vi "Write 7z config.vi"(8 "error in (no error)":errorcluster, 11 "PostBuildSupport in":refnum<class "PostBuildSupport.lvclass">) -> (0 "error out":errorcluster, 3 "PostBuildSupport out":refnum<class "PostBuildSupport.lvclass">)   [LabVIEW 2019, in "PostBuildSupport.lvclass"]
uses:
  PostBuildSupport.lvclass
  PostBuildSupport.lvclass/PostBuildSupport.ctl
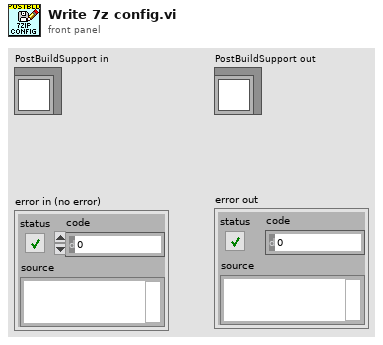
[diagram p1: front panel]
types:
  T1 = enum16{"open", "replace", "create", "open or create", "replace or create", "replace or create with confirmation"}
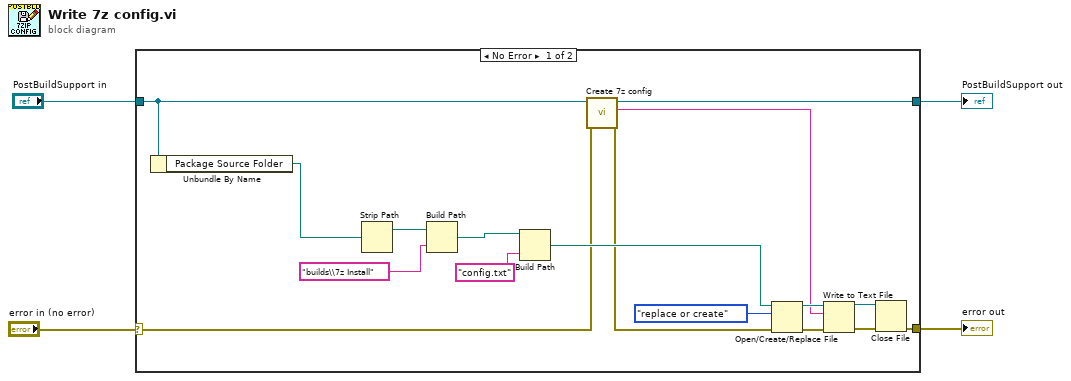
[diagram p0: block diagram]
diagram:
  n1 = case shown="No Error" "error in (no error)" {
    selector: "error in (no error)" -> [w9 w22]
    tunnel: [w13 w22] -> w4
    tunnel: "PostBuildSupport in" -> [w5 w23]
    tunnel: [w6 w23] -> w2
    frame No Error {
      n2 = Unbundle By Name(w5) -> ("Package Source Folder"=w10:path)
      n3 = Strip Path(path=w10) -> (stripped path=w20:path)  [unwired: 1 out]
      n4 = Build Path(base path=w20, name or relative path="builds\\7z Install") -> (appended path=w12:path)
      n5 = Build Path(base path=w12, name or relative path="config.txt") -> (appended path=w17:path)
      n6 = call "Create 7z config.vi"("error in (no error)"=w9, "PostBuildSupport in"=w5) -> ("error out"=w8:errorcluster, "resulting string"=w7:string, "PostBuildSupport out"=w6:refnum<class "PostBuildSupport.lvclass">)  [unwired: 7 in]
      n7 = Open/Create/Replace File(file path (use dialog)=w17, error in=w8, operation (0:open)=T1."replace or create") -> (refnum out=w19:refnum<file>, error out=w18:errorcluster)  [unwired: 3 in, 1 out]
      n8 = Write to Text File(file (use dialog)=w19, text=w7, error in=w18) -> (refnum out=w14:refnum<file>, error out=w15:errorcluster)  [unwired: 1 in, 1 out]
      n9 = Close File(refnum=w14, error in=w15) -> (error out=w13:errorcluster)  [unwired: 1 out]
    }
    frame Error {
    }
  }
  "error out" <- w4
  "PostBuildSupport out" <- w2
